vi "Create.vi"(5 "Collection Contains in":refnum<class "Collection Contains.lvclass">, 8 "error in (no error)":errorcluster, 11 "Item":variant) -> (0 "error out":errorcluster, 3 "Collection Contains":refnum<class "Collection Contains.lvclass">)   [LabVIEW 2017, in "Transparent Assertions.lvlib" / "Collection Contains.lvclass"]
uses:
  Collection Contains.lvclass
  Collection Contains.lvclass/Collection Contains.ctl
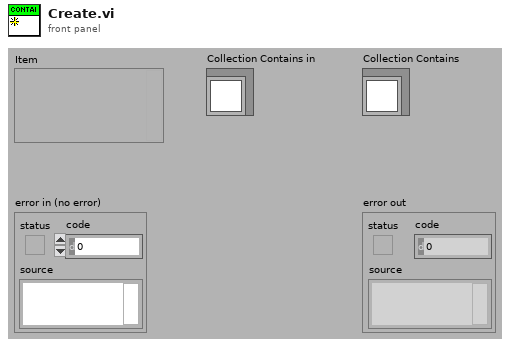
[diagram p1: front panel]
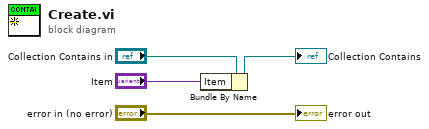
[diagram p0: block diagram]
diagram:
  n1 = Bundle By Name(cluster="Collection Contains in", "Item"="Item") -> (→"Collection Contains":refnum<class "Collection Contains.lvclass">)
  "error out" <- "error in (no error)"
